vi "ShooterMain.vi"(6 "Invert?":bool, 8 "Boolean2":bool, 9 "Boolean1":bool, 10 "Input":dbl, 11 "Mode":enum16{"Open", "Control", "PID Control"}(ring)) -> (2 "Output":dbl)   [LabVIEW 2016]
uses:
  <vilib>/Rock Robotics/SystemInterfaces/DIO/FPGA_DIOPWMChannel.ctl
  <vilib>/Rock Robotics/WPI/MotorControl/WPI_MotorControlOpen VictorSP.vi
  <vilib>/addons/control/pid/pid.llb/PID (DBL).vi
  <vilib>/addons/control/pid/NI_PID_pid.lvlib
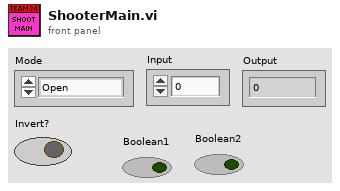
[diagram p1: front panel]
types:
  T1 = typedef "FPGA_DIOPWMChannel.ctl" = enum8{"PWM 0", "PWM 1", "PWM 2", "PWM 3", "PWM 4", "PWM 5", "PWM 6", "PWM 7", "PWM 8", "PWM 9", "PWM MXP 0", "PWM MXP 1", "PWM MXP 2", "PWM MXP 3", "PWM MXP 4", "PWM MXP 5", "PWM MXP 6", "PWM MXP 7", "PWM MXP 8", "PWM MXP 9", "Invalid"}
  T2 = typedef "WPI_MotorControlDeviceRef.ctl" = cluster{"DeviceStatus":errorcluster, "Type":T3, "PWM":cluster{"PWM Channel":T1, "DeadBand":T4}, "CAN":cluster{"Device Number":u8, "SetOutput VI Ref":variant, "GetOutput VI Ref":variant, "Enable VI Ref":variant, "Disable VI Ref":variant, "Data":variant}, "Invert":bool}
  T3 = typedef "WPI_MotorControlType.ctl" = enum16{"PWM", "CAN"}
  T4 = typedef "WPI_PWMDeadband.ctl" = cluster{"Name":string, "maxPositivePwm":i32, "minPositivePwm":i32, "centerPwm":i32, "maxNegativePwm":i32, "minNegativePwm":i32, "angularRange":u16}
  T5 = cluster{"proportional gain (Kc)":dbl, "integral time (Ti, min)":dbl, "derivative time (Td, min)":dbl}
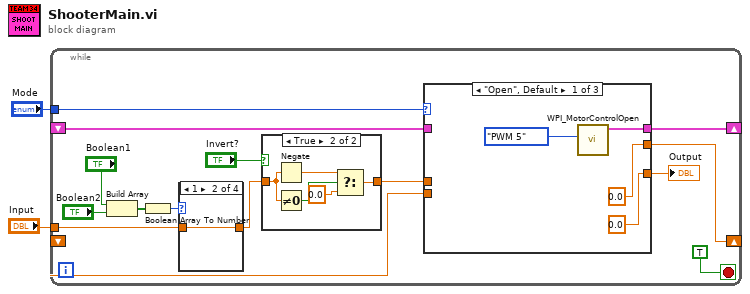
[diagram p0: block diagram]
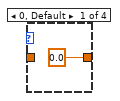
[diagram p2: hidden frame]
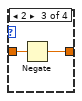
[diagram p3: hidden frame]
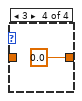
[diagram p4: hidden frame]
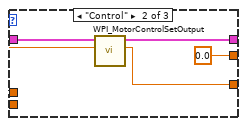
[diagram p6: hidden frame]
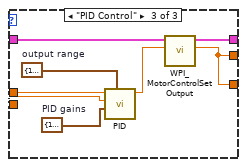
[diagram p7: hidden frame]
diagram:
  n1 = while {
    tunnel: "Mode" -> [w16]
    shift-right: [w15] -> _
    shift-left: _ -> [w14]
    tunnel: "Input" -> [w4]
    shift-right: [w11] -> _
    shift-left: _ -> [w10]
    stop <- TRUE stop-if-true
    n2 = Build Array("Boolean1", "Boolean2") -> (w6:bool[])
    n3 = Boolean Array To Number(Boolean array=w6) -> (number=w5:u32)
    n4 = case shown="1" w5 {
      tunnel: [0.0 ("Input") w19 w20 0.0 ("Input")] -> w3
      tunnel: w4 -> [_ w19 w21 _]
      frame 0, Default {
      }
      frame 1 {
      }
      frame 2 {
        n5 = Negate(x=w21) -> (-x=w20:dbl)
      }
      frame 3 {
      }
    }
    n6 = case shown="True" "Invert?" {
      tunnel: [w23 w25] -> w13
      tunnel: w3 -> [w23 w24]
      frame False {
      }
      frame True {
        n7 = Negate(x=w24) -> (-x=w27:dbl)
        n8 = Not Equal To 0?(x=w24) -> (x != 0?=w28:bool)
        n9 = Select(t=w27, s=w28, f=0.0) -> (s? t:f=w25:dbl)
      }
    }
    n10 = case shown="\"Open\", Default" w16 {
      tunnel: [w32 w36 w42] -> w15
      tunnel: w14 -> [_ w37 w43]
      tunnel: w13 -> [_ w34 w44]
      tunnel: [0.0 ("Motor Output") 0.0 ("Motor Output") w39] -> w11
      tunnel: w10 -> [_ _ w40]
      tunnel: [0.0 ("Motor Output") w33 w39] -> w9
      frame "Open", Default {
        n11 = call-poly <vilib>:"WPI_MotorControlOpen.vi"("PWM Channel"=FPGA_DIOPWMChannel."PWM 5") -> ("MotorControlDeviceRef"=w32:T2)  [unwired: 9 in, 1 out]
      }
      frame "Control" {
        n12 = call <vilib>:"WPI_MotorControlSetOutput.vi"("Output"=w34, "MotorControlDevRef"=w37) -> ("Motor Output"=w33:dbl, "MotorControlDevRef"=w36:T2)  [unwired: 7 in, 1 out]
      }
      frame "PID Control" {
        w38 = T5 {"proportional gain (Kc)"=1.0, "integral time (Ti, min)"=0.01, "derivative time (Td, min)"=0.0}  # PID gains
        w45 = cluster{"output high":dbl, "output low":dbl} {"output high"=1.0, "output low"=-1.0}  # output range
        n13 = call-poly <vilib>:"PID.vi"("output range"=w45, "PID gains"=w38, "process variable"=w40, "setpoint"=w44) -> ("output"=w41:dbl)  [unwired: 6 in, 1 out]
        n14 = call <vilib>:"WPI_MotorControlSetOutput.vi"("Output"=w41, "MotorControlDevRef"=w43) -> ("Motor Output"=w39:dbl, "MotorControlDevRef"=w42:T2)  [unwired: 7 in, 1 out]
      }
    }
    "Output" <- w9
  }
